vi "3_2.vi"() -> ()   [LabVIEW 2018]
panel:
  out "X(i-3)":i32
  out "X(i-2)":i32
  out "X(i-1)":i32
  out "X(i)":i32
  in  "stop":bool
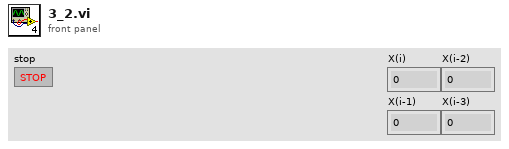
[diagram p1: front panel]
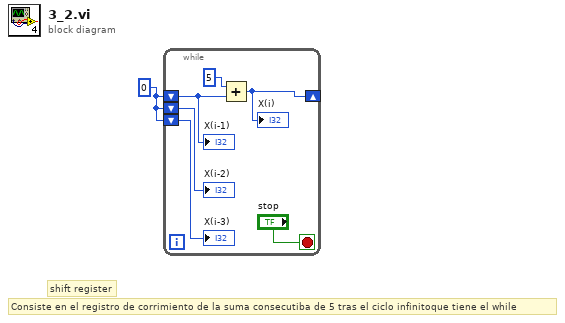
[diagram p0: block diagram]
diagram:
  w1 = 0 ("x")
  # "shift register"
  # "Consiste en el registro de corrimiento de la suma consecutiba de 5 tras el ciclo infinitoque tiene el while"
  n1 = while {
    shift-right: [w5] -> _
    shift-left: w1 -> [w4]
    shift-left: w1 -> [w3]
    shift-left: w1 -> [w2]
    stop <- "stop" stop-if-true
    n2 = Add(x=5, y=w4) -> (x+y=w5:i32)
    "X(i)" <- w5
    "X(i-1)" <- w4
    "X(i-2)" <- w3
    "X(i-3)" <- w2
  }
